vi "GetParam.vi"(8 "error in (no error)":errorcluster caption="entrée d'erreur (pas d'erreur)", 11 "Manhattan_distances.lvclass":refnum<class "Manhattan_distances.lvclass">) -> (0 "error out":errorcluster caption="sortie d'erreur", 2 "manhattan_distances":cluster{"sum_over_features":bool}={"sum_over_features"=TRUE}, 3 "Manhattan_distances.lvclass":refnum<class "Manhattan_distances.lvclass">)   [LabVIEW 2020, in "Manhattan_distances.lvclass"]
doc: "Get Parameters"
uses:
  Manhattan_distances.lvclass
  Manhattan_distances.lvclass/Manhattan_distances.ctl
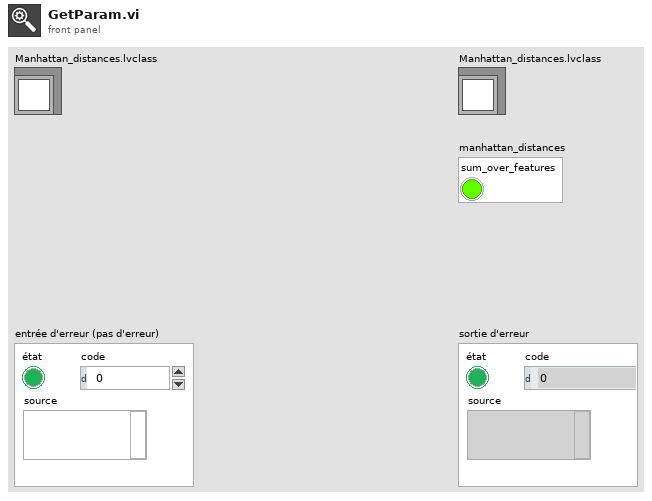
[diagram p1: front panel]
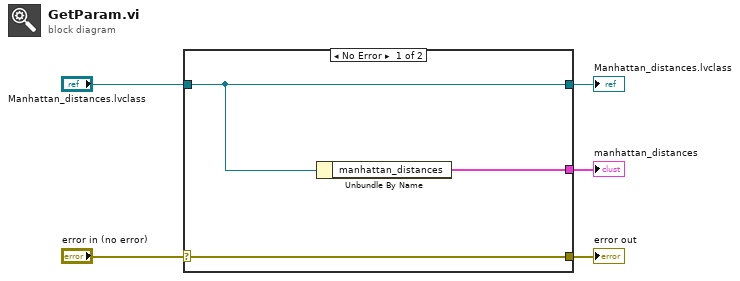
[diagram p0: block diagram]
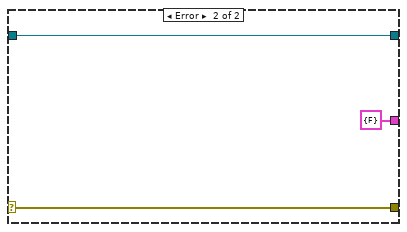
[diagram p2: hidden frame]
diagram:
  n1 = case shown="No Error" "error in (no error)" {
    selector: "error in (no error)" -> [w8 w10]
    tunnel: [w8 w10] -> w4
    tunnel: [w7 w11] -> w2
    tunnel: "Manhattan_distances.lvclass" -> [w7 w11]
    tunnel: [w6 cluster{"sum_over_features":bool} {"sum_over_features"=FALSE} ("manhattan_distances")] -> w1
    frame No Error {
      n2 = Unbundle By Name(w7) -> ("manhattan_distances"=w6:cluster{"sum_over_features":bool})
    }
    frame Error {
    }
  }
  "error out" <- w4
  "Manhattan_distances.lvclass" <- w2
  "manhattan_distances" <- w1
